vi "NI VeriStand - Set Custom Device Channel Value Table.vi"(8 "error in (no error)":errorcluster, 9 "Values":dbl[](array[numeric]), 10 "Names":string[](array[string]), 11 "Channel Ref in":T1 format="%.0x") -> (0 "error out":errorcluster, 3 "Channel Ref out":T1=18446744073709551615 format="%.0x")   [LabVIEW 2020, in "Custom Device API.lvlib"]
uses:
  <vilib>/NI VeriStand/Custom Device API/Custom Device API.lvlib
  <vilib>/NI VeriStand/Custom Device API/Custom Device Item Ref.ctl
  NationalInstruments.VeriStand.SystemStorage
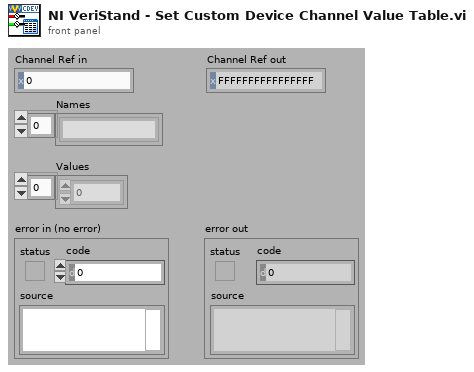
[diagram p1: front panel]
types:
  T1 = typedef "Custom Device API.lvlib/Custom Device Item Ref.ctl" = u64
  T2 = typedef "Custom Device API.lvlib/Custom Device Pointer.ctl" = refnum<k24>
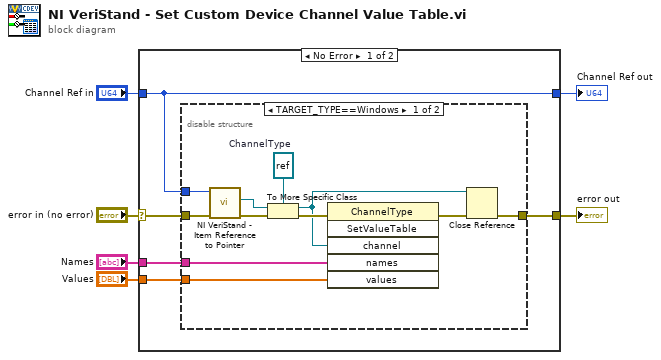
[diagram p0: block diagram]
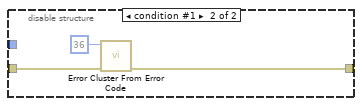
[diagram p2: hidden frame]
diagram:
  n1 = case shown="No Error" "error in (no error)" {
    selector: "error in (no error)" -> [w11 w27]
    tunnel: [w9 w27] -> w6
    tunnel: "Channel Ref in" -> [w10 w26]
    tunnel: [w10 w26] -> w4
    tunnel: "Names" -> [w8 _]
    tunnel: "Values" -> [w7 _]
    frame No Error {
      n2 = disable-structure shown="TARGET_TYPE==Windows" {
        disable-tunnel: w11 -> [w21 w25]
        disable-tunnel: w10 -> [w20 _]
        disable-tunnel: [w18 w24] -> w9
        disable-tunnel: w8 -> [w13 _]
        disable-tunnel: w7 -> [w14 _]
        frame condition #0 (active) {
          w17 = refnum<k24> refnum  # ChannelType
          n3 = call <vilib>:"NI VeriStand - Item Reference to Pointer.vi"("error in (no error)"=w21, "Item Ref in"=w20) -> ("error out"=w15:errorcluster, "Node Pointer"=w16:T2)  [unwired: 6 in, 2 out]
          n4 = To More Specific Class(target class=w17, reference=w16, error in=w15) -> (specific class reference=w12:refnum<k24>, error out=w22:errorcluster)
          n5 = invoke class="ChannelType" method="SetValueTable"(error in=w22, "channel"=w12, "names"=w13, "values"=w14) -> (error out=w19:errorcluster)  [unwired: 2 in, 5 out]
          n6 = Close Reference(reference=w12, error in (no error)=w19) -> (error out=w18:errorcluster)
        }
        frame condition #1 {
          n7 = call <vilib>:"Error Cluster From Error Code.vi"("error in (no error)"=w25, "error code (0)"=36) -> ("error out"=w24:errorcluster)  [unwired: 7 in]
        }
      }
    }
    frame Error {
    }
  }
  "error out" <- w6
  "Channel Ref out" <- w4
